vi "Find FlatSequence.vi"(8 "error in (no error)":errorcluster, 9 "i in":i32, 11 "VI in":refnum<vi>) -> (0 "error out":errorcluster, 1 "i out":i32, 3 "FlatSequences":T1[](array[typedef]))   [LabVIEW 2023, in "VIDoc Parsing.lvlib" / "Structure Reporter.lvlib"]
uses:
  Structure Reporter.lvlib
  Structure Result 2.ctl
  <vilib>/Utility/traverseref.llb/TRef TravTarget.ctl
  <vilib>/Utility/traverseref.llb/VI Scripting - Traverse.lvlib
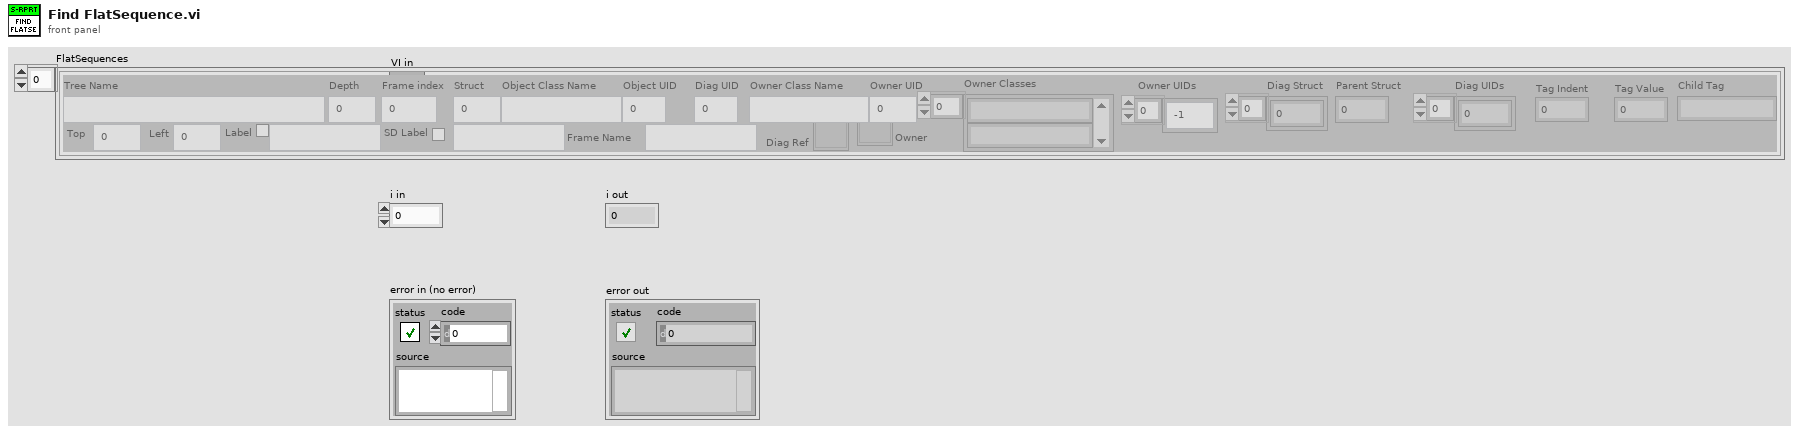
[diagram p1: front panel]
types:
  T1 = typedef "VIDoc Parsing.lvlib/Structure Reporter.lvlib/Structure Result 2.ctl" = cluster{"Depth":i32, "Top":i32, "Left":i32, "Frame index":i32, "Struct":i32, "Object Class Name":string, "Object UID":i32, "Label Visible":bool, "Object Label":string, "SD Label Visible":bool, "Object SD Label":string, "Frame Name":string, "Diag UID":i32, "Owner Class Name":string, "Owner UID":i32, "Diag Struct":i32[], "Parent Struct":i32, "Diag UIDs":i32[], "Tree Name":string, "Diag Ref":refnum<vi>, "Owner Classes":string[], "Owner":refnum<vi>, "Owner UIDs":i32[], "Tag Indent":i32, "Tag Value":i32, "Child Tag":string}
  T2 = typedef "TRef TravTarget.ctl" = enum16{"FP", "BD", "Other"}
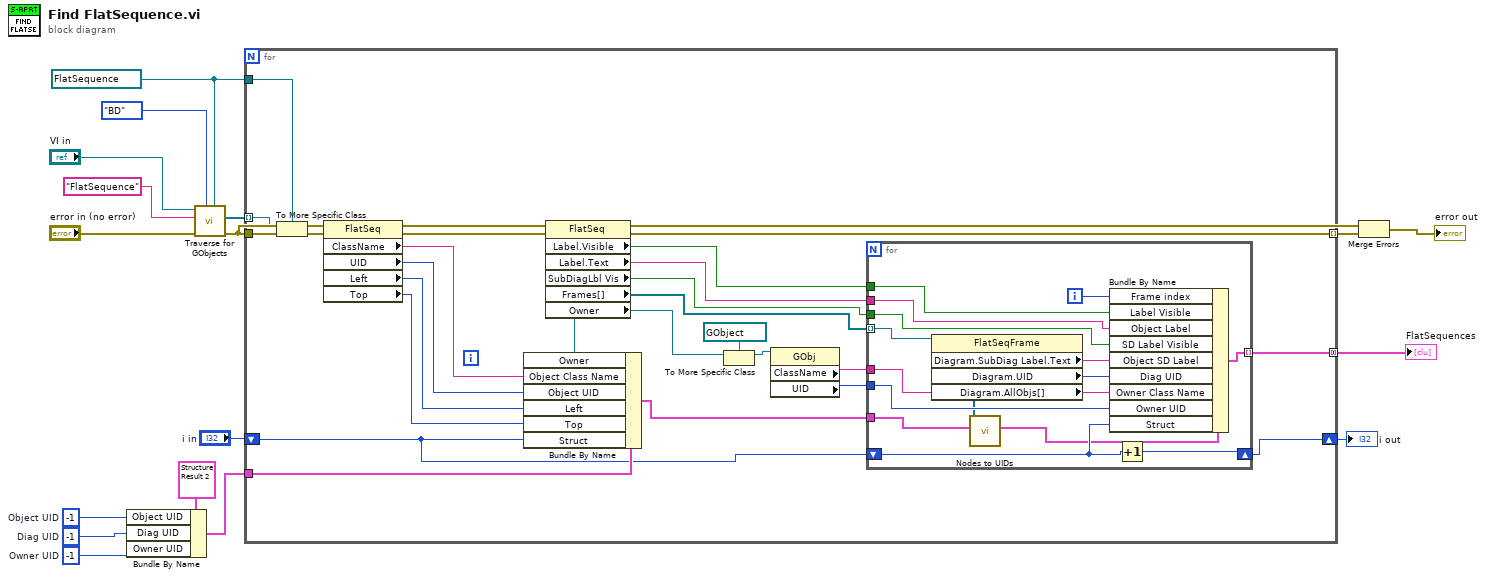
[diagram p0: block diagram]
diagram:
  w3 = -1  # Owner UID
  w4 = -1  # Diag UID
  w5 = -1  # Object UID
  w14 = refnum<vi> refnum ("Other Refnum")
  n1 = Bundle By Name(cluster=T1 {"Depth"=0, "Top"=0, "Left"=0, "Frame index"=0, "Struct"=0, "Object Class Name"="", "Object UID"=0, "Label Visible"=FALSE, "Object Label"="", "SD Label Visible"=FALSE, "Object SD Label"="", "Frame Name"="", "Diag UID"=0, "Owner Class Name"="", "Owner UID"=0, "Diag Struct"=[], "Parent Struct"=0, "Diag UIDs"=[], "Tree Name"="", "Diag Ref"=refnum, "Owner Classes"=[], "Owner"=refnum, "Owner UIDs"=[], "Tag Indent"=0, "Tag Value"=0, "Child Tag"=""}, "Object UID"=w5, "Diag UID"=w4, "Owner UID"=w3) -> (w2:T1)
  n2 = call <vilib>:"Traverse for GObjects.vi"("Other Refnum"=w14, "Traverse Target"=TRef_TravTarget."BD", "error in (no error)"="error in (no error)", "Class Name"="FlatSequence", "VI Refnum"="VI in") -> ("error out"=w1:errorcluster, "References"=w13:refnum<vi>[])  [unwired: 3 in, 2 out]
  n3 = for {
    tunnel: w13 -> [w41] mode=indexing
    tunnel: w14 -> [w40]
    tunnel: w2 -> [w39]
    tunnel: [w24] -> w15 mode=concatenating
    tunnel: w1 -> [w23]
    tunnel: [w21] -> w17 mode=indexing
    shift-right: [w19] -> w7
    shift-left: "i in" -> [w20]
    n4 = To More Specific Class(target class=w40, reference=w41, error in=w23) -> (specific class reference=w42:refnum<vi>, error out=w43:errorcluster)
    n5 = property class="FlatSeq"(reference=w42, error in=w43) -> (reference out=w26:refnum<vi>, error out=w22:errorcluster, "ClassName"=w38:string, "UID"=w37:i32, "Left"=w36:i32, "Top"=w35:i32)
    n6 = property class="FlatSeq"(reference=w26, error in=w22) -> (error out=w21:errorcluster, "Label.Visible"=w34:bool, "Label.Text"=w29:string, "SubDiagLbl Vis"=w28:bool, "Frames[]"=w27:refnum<vi>[], "Owner"=w18:refnum<vi>)  [unwired: 1 out]
    n7 = Bundle By Name(cluster=w39, "Owner"=w18, "Object Class Name"=w38, "Object UID"=w37, "Left"=w36, "Top"=w35, "Struct"=w20) -> (w25:T1)
    n8 = To More Specific Class(target class=refnum<vi> refnum ("Other Refnum"), reference=w18) -> (specific class reference=w32:refnum<vi>)  [unwired: 1 in, 1 out]
    n9 = property class="GObj"(reference=w32) -> ("ClassName"=w31:string, "UID"=w30:i32)  [unwired: 1 in, 2 out]
    n10 = for {
      tunnel: w34 -> [w58]
      tunnel: w31 -> [w53]
      tunnel: w30 -> [w52]
      tunnel: w29 -> [w57]
      tunnel: w28 -> [w56]
      tunnel: [w51] -> w24 mode=indexing
      tunnel: w27 -> [w50] mode=indexing
      tunnel: w25 -> [w45]
      shift-right: [w47] -> w19
      shift-left: w20 -> [w48]
      i -> [w49]
      n11 = property class="FlatSeqFrame"(reference=w50) -> ("Diagram.SubDiag Label.Text"=w55:string, "Diagram.UID"=w54:i32, "Diagram.AllObjs[]"=w46:refnum<vi>[])  [unwired: 1 in, 2 out]
      n12 = call "Nodes to UIDs.vi"("cluster"=w45, "All Objects[]"=w46) -> ("Nodes"=w44:T1)  [unwired: 9 in]
      n13 = Bundle By Name(cluster=w44, "Frame index"=w49, "Label Visible"=w58, "Object Label"=w57, "SD Label Visible"=w56, "Object SD Label"=w55, "Diag UID"=w54, "Owner Class Name"=w53, "Owner UID"=w52, "Struct"=w48) -> (w51:T1)
      n14 = Increment(x=w48) -> (x+1=w47:i32)
    }
  }
  "FlatSequences" <- w15
  "i out" <- w7
  n15 = Merge Errors(w1, w17) -> (→"error out":errorcluster)
